vi "SetReset.vi"(8 "error in (no error)":errorcluster, 9 "SequenceNumber":u32, 10 "address":u32, 11 "connection ID":refnum<k16>) -> (0 "error out":errorcluster, 1 "SequenceNumber out":i32, 2 "Address out":u32, 3 "connection ID out":refnum<k16>)   [LabVIEW 2009]
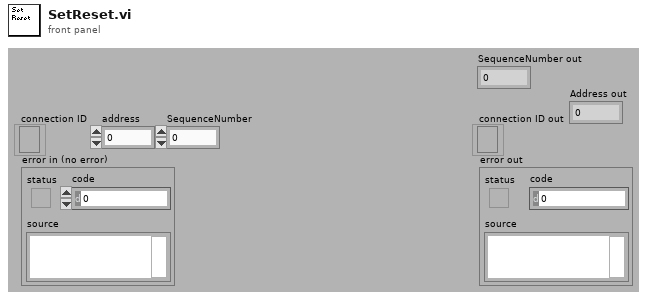
[diagram p1: front panel]
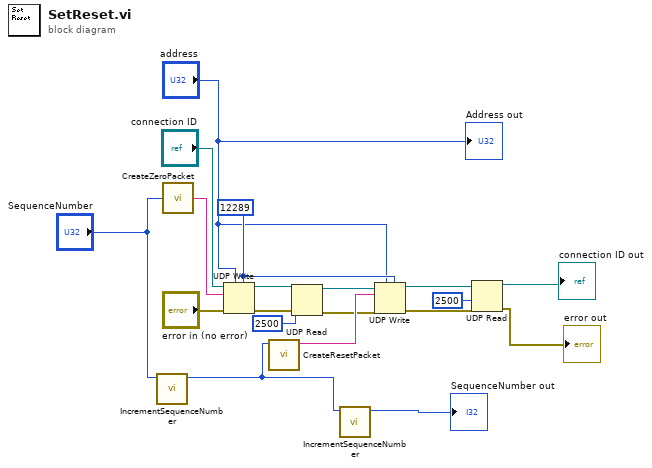
[diagram p0: block diagram]
diagram:
  w15 = u16 12289 ("port or service name")
  n1 = call "IncrementSequenceNumber.vi"("In"="SequenceNumber") -> ("Out"=w14:i32)  [unwired: 10 in]
  n2 = call "CreateZeroPacket.vi"("SequenceNumber"="SequenceNumber") -> ("ZeroPacket"=w16:string)
  n3 = UDP Write(address="address", port or service name=w15, connection ID="connection ID", data in=w16, 8:"error in (no error)") -> (error out=w8:errorcluster, 3:w10:refnum<k16>)  [unwired: 1 in]
  n4 = call "CreateResetPacket.vi"("SequenceNumber"=w14) -> ("ResetPacket"=w11:string)  [unwired: 10 in]
  n5 = UDP Read(connection ID=w10, timeout ms (25000)=2500, 8:w8) -> (error out=w7:errorcluster, 3:w9:refnum<k16>)  [unwired: 1 in, 3 out]
  n6 = call "IncrementSequenceNumber.vi"("In"=w14) -> ("Out"=→"SequenceNumber out":i32)  [unwired: 10 in]
  n7 = UDP Write(address="address", port or service name=w15, connection ID=w9, data in=w11, 8:w7) -> (error out=w4:errorcluster, 3:w5:refnum<k16>)  [unwired: 1 in]
  n8 = UDP Read(connection ID=w5, timeout ms (25000)=2500, 8:w4) -> (error out=→"error out":errorcluster, 3:→"connection ID out":refnum<k16>)  [unwired: 1 in, 3 out]
  "Address out" <- "address"
